vi "ConfigDlg.vi"(8 "error in (no error)":errorcluster, 11 "SaveWaveforms in":refnum<class "SaveWaveforms.lvclass">) -> (0 "error out":errorcluster, 2 "Changed":bool, 3 "SaveWaveforms out":refnum<class "SaveWaveforms.lvclass">)   [LabVIEW 2018, in "AnalysisPlugins.lvlib" / "SaveWaveforms.lvclass"]
uses:
  SaveWaveforms.lvclass
  X:/Projects/PMUCal/Modules/Analysis/AnalysisPlugins/AnalysisPluginBaseClass/AnalysisPluginsBase.lvclass
  C:/Program Files (x86)/National Instruments/LabVIEW 2018/user.lib/NIST/BaseClasses/BasePlugin_class/BasePlugin.lvclass
  AnalysisPluginBaseClass/AnalysisPluginsBase.lvclass/AnalysisPluginsBase.ctl
  <userlib>/NIST/BaseClasses/BasePlugin_class/BasePlugin.lvclass/BasePlugin.ctl
  AnalysisPluginBaseClass/Accessors/Read Duration.vi
  <userlib>/NIST/BaseClasses/BasePlugin_class/Accessors/Read PluginIniFilePath.vi
  AnalysisPluginBaseClass/Accessors/Write Duration.vi
  <vilib>/Utility/config.llb/NI_LVConfig.lvlib
panel:
  in  "BtnCancel":bool
  in  "btnDone":bool
  in  "Duration":dbl
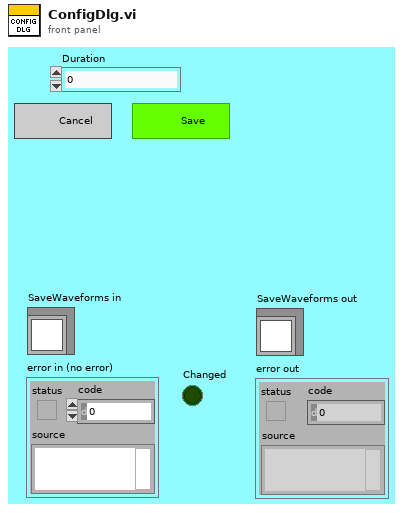
[diagram p1: front panel]
types:
  T1 = enum32{"Invalid", "Standard", "Closed", "Hidden", "Minimized", "Maximized"}
  T2 = enum32{"Invalid", "Default", "Floating", "Floating/Auto-Hide", "Modal"}
  T3 = typedef "NI_LVConfig.lvlib/Config Data RefNum.ctl" = refnum<k1>
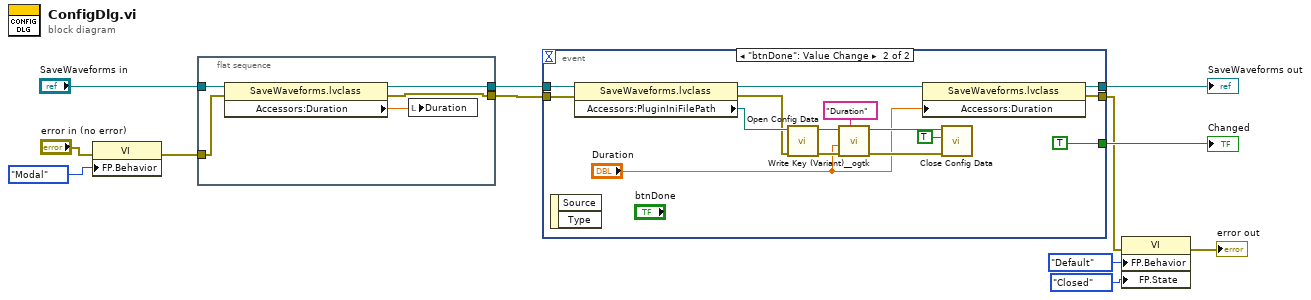
[diagram p0: block diagram]
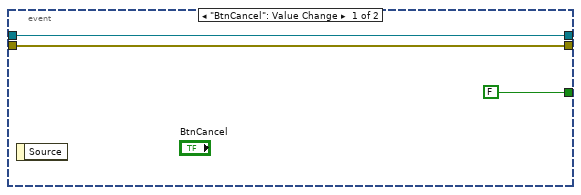
[diagram p2: hidden frame]
diagram:
  n1 = property class="VI"(error in="error in (no error)", "FP.Behavior"=T2."Modal" ("Front Panel Window:Behavior")) -> (error out=w9:errorcluster)  [unwired: 1 in, 1 out]
  n2 = flat-sequence {
    tunnel: "SaveWaveforms in" -> [w17]
    tunnel: w9 -> [w15]
    tunnel: [w14] -> w7
    tunnel: [w13] -> w8
    frame #0 {
      n3 = property class="SaveWaveforms.lvclass"(reference=w17, error in=w15) -> (reference out=w13:refnum<class "SaveWaveforms.lvclass">, error out=w14:errorcluster, "Accessors:Duration"=w16:dbl)
      n4 = local write "Duration"(w16) -> ()
    }
  }
  n5 = event shown="[1] \"btnDone\": Value Change" {
    selector: _ -> [_ _]
    dyn-events: _ -> [_ _]
    timeout: _ -> [_ _]
    tunnel: w8 -> [w19 w35]
    tunnel: [w20 w25] -> w2
    tunnel: w7 -> [w20 w34]
    tunnel: [w19 w21] -> w6
    tunnel: [FALSE TRUE] -> w5
    event "BtnCancel": Value Change {
      n6 = event-data() -> ()  [unwired: 1 in, 1 out]
    }
    event "btnDone": Value Change {
      n7 = event-data() -> ()  [unwired: 1 in, 2 out]
      n8 = property class="SaveWaveforms.lvclass"(reference=w35, error in=w34) -> (reference out=w24:refnum<class "SaveWaveforms.lvclass">, error out=w32:errorcluster, "Accessors:PluginIniFilePath"=w33:path)
      n9 = call <vilib>:"Open Config Data.vi"("error in (no error)"=w32, "configuration file path"=w33) -> ("error out"=w31:errorcluster, "refnum"=w30:T3)  [unwired: 7 in, 1 out]
      n10 = call <userlib>:"Write Key (Variant)__ogtk.vi"("section"="Duration", "error in (no error)"=w31, "key-value"="Duration", "refnum"=w30) -> ("error out"=w28:errorcluster, "refnum out"=w27:T3)  [unwired: 6 in]
      n11 = property class="SaveWaveforms.lvclass"(reference=w24, "Accessors:Duration"="Duration") -> (reference out=w21:refnum<class "SaveWaveforms.lvclass">, error out=w25:errorcluster)  [unwired: 1 in]
      n12 = call <vilib>:"Close Config Data.vi"("error in (no error)"=w28, "write file if changed (T)"=TRUE, "refnum"=w27) -> ()  [unwired: 7 in, 2 out]
    }
  }
  "SaveWaveforms out" <- w6
  "Changed" <- w5
  n13 = property class="VI"(error in=w2, "FP.Behavior"=T2."Default" ("Front Panel Window:Behavior"), "FP.State"=T1."Closed" ("Front Panel Window:State")) -> (error out=→"error out":errorcluster)  [unwired: 1 in, 1 out]
